vi "OEE_calculate_targets.vi"(8 "error_in":errorcluster) -> (0 "error_out":errorcluster)   [LabVIEW 2019]
uses:
  FGV/SQL_raw_data/FGV_OEE_SQL_raw_data.ctl
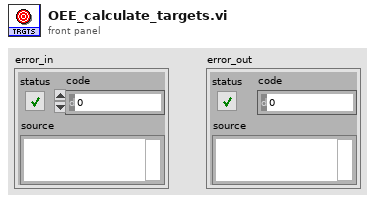
[diagram p1: front panel]
types:
  T1 = typedef "FGV_OEE_SQL_raw_data.ctl" = enum16{"initialize", "set_reference_name", "set_timestamp", "set_OK_NOK_count", "set_config_info", "set_pace", "set_availability", "set_hourly_ok_count", "set_targets", "get_all_info"}
  T2 = typedef "OEE_SQL_raw_data.ctl" = cluster{"reference_name":string, "data_timestamp":timestamp, "OK_NOK_count":string[][], "config_info":string[], "pace":string[][], "availability":string[], "hourly_ok_count":string[][], "shift_number":i8, "shift_start":i8, "shift_end":i8, "TAKT":u16, "FTTH_target":u16, "BOTTLENECK_station":string, "targets_hourly":u16[], "target_shift":u16}
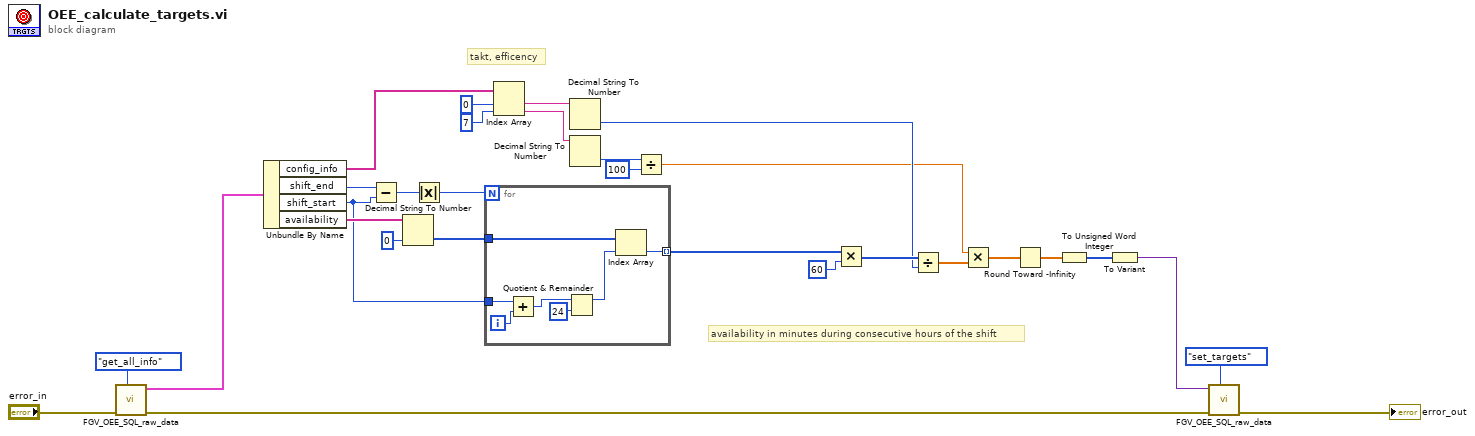
[diagram p0: block diagram]
diagram:
  # "takt, efficency"
  # "availability in minutes during consecutive hours of the shift"
  n1 = call "FGV_OEE_SQL_raw_data.vi"("options"=FGV_OEE_SQL_raw_data."get_all_info", "error_in"="error_in") -> ("error_out"=w1:errorcluster, "SQL_raw_data_out"=w28:T2)  [unwired: 8 in]
  n2 = Unbundle By Name(w28) -> ("config_info"=w20:string[], "shift_end"=w24:i8, "shift_start"=w21:i8, "availability"=w27:string[])
  n3 = Subtract(x=w24, y=w21) -> (x-y=w23:i8)
  n4 = Decimal String To Number(string=w27, default (0L)=u16 0 ("default (0 I32)")) -> (number=w25:u16[])  [unwired: 1 in, 1 out]
  n5 = Absolute Value(x=w23) -> (abs(x)=w22:i8)
  n6 = for {
    N: w22 -> [_]
    tunnel: w25 -> [w37]
    tunnel: w21 -> [w33]
    tunnel: [w34] -> w13 mode=indexing
    i -> [w32]
    n7 = Add(x=w33, y=w32) -> (x+y=w31:i32)
    n8 = Quotient & Remainder(x=w31, y=i8 24) -> (x-y*floor(x/y)=w35:i32)  [unwired: 1 out]
    n9 = Index Array(array=w37, index=w35) -> (element=w34:u16)
  }
  n10 = Index Array(array=w20, index #1=0 ("index"), index #2=7 ("index")) -> (element #1=w17:string, element #2=w16:string)
  n11 = Decimal String To Number(string=w17) -> (number=w10:i32)  [unwired: 2 in, 1 out]
  n12 = Decimal String To Number(string=w16) -> (number=w15:i32)  [unwired: 2 in, 1 out]
  n13 = Divide(x=w15, y=100) -> (x/y=w8:dbl)
  n14 = Multiply(x=w13, y=60) -> (x*y=w11:i32[])
  n15 = Divide(x=w11, y=w10) -> (x/y=w9:dbl[])
  n16 = Multiply(x=w8, y=w9) -> (x*y=w7:dbl[])
  n17 = Round Toward -Infinity(1:w7) -> (0:w6:dbl[])
  n18 = To Unsigned Word Integer(number=w6) -> (unsigned 16bit integer=w4:u16[])
  n19 = To Variant(anything=w4) -> (Variant=w3:variant)
  n20 = call "FGV_OEE_SQL_raw_data.vi"("options"=FGV_OEE_SQL_raw_data."set_targets", "error_in"=w1, "input"=w3) -> ("error_out"=→"error_out":errorcluster)  [unwired: 7 in, 1 out]
